vi "Queue Manager.vi"(0 "queue in":refnum<queue>, 5 "Queue States In":cluster{"Enum":T1, "Data":variant}[](array[cluster])=[{"Enum"=enum."Read GUI Pars", "Data"=variant}], 9 "Place New Element":enum16{"Back", "Front", "Replace"}(ring), 11 "Error IN":errorcluster, 12 "Ignore Errors":bool) -> (4 "queue out":refnum<queue>, 8 "Last Error":errorcluster, 15 "Error OUT":errorcluster)   [LabVIEW 2016]
uses:
  Types/State Control.ctl
  Types/Global Variables.vi
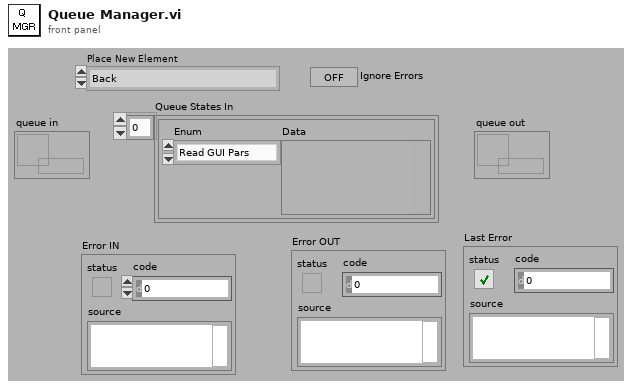
[diagram p1: front panel]
types:
  T1 = typedef "State Control.ctl" = enum16{"Startup", "Read Config File", "Initilize Optional Hardware", "Idle", "New Session", "Read GUI Pars", "Configure Hardware", "Initialize Set", "Pre-Scan", "Scan", "Post-Scan", "Exit Set", "Automated Tuning", "Manual Tuning", "Check Calibration", "Optimize RF Power", "Test Scan", "Set Oxy QA-Scan Pars", "Find Peaks", "Update from Cursors", "Flag Bad Set", "Mark transition time", "Measure Q", "Measure Noise", "Rotate Magnet", "Lock Field", "Engineering Tuning", "Zero Voltages", "Update Center Field", "Refit Data", "Open Session Data Folder", "AfterSave", "Undo Auto Update Pars", "Read from Script", "End Session", "Quit Software", "Error"}
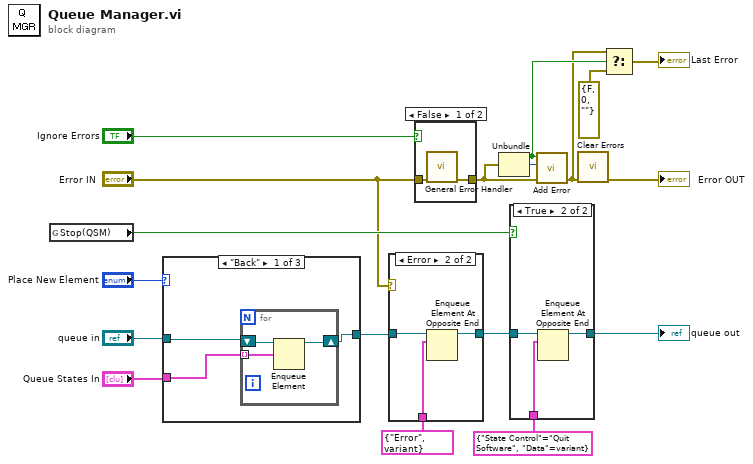
[diagram p0: block diagram]
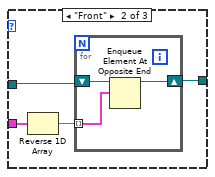
[diagram p5: hidden frame]
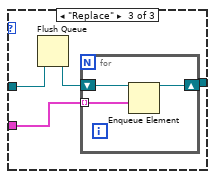
[diagram p6: hidden frame]
diagram:
  n1 = global read "Global Variables.vi" "Stop(QSM)"() -> (w10:bool)
  n2 = case shown="\"Back\"" "Place New Element" {
    tunnel: "Queue States In" -> [w19 w28 w33]
    tunnel: "queue in" -> [w21 w26 w35]
    tunnel: [w20 w25 w32] -> w17
    frame "Back" {
      n3 = for {
        shift-right: [w23] -> w20
        shift-left: w21 -> [w24]
        tunnel: w19 -> [w22] mode=indexing
        n4 = Enqueue Element(queue=w24, element=w22) -> (queue out=w23:refnum<queue>)  [unwired: 2 in, 2 out]
      }
    }
    frame "Front" {
      n5 = Reverse 1D Array(array=w28) -> (reversed array=w27:cluster{"Enum":T1, "Data":variant}[])
      n6 = for {
        tunnel: w27 -> [w30] mode=indexing
        shift-right: [w29] -> w25
        shift-left: w26 -> [w31]
        n7 = Enqueue Element At Opposite End(queue=w31, element=w30) -> (queue out=w29:refnum<queue>)  [unwired: 2 in, 2 out]
      }
    }
    frame "Replace" {
      n8 = Flush Queue(queue=w35) -> (queue out=w34:refnum<queue>)  [unwired: 1 in, 2 out]
      n9 = for {
        tunnel: w33 -> [w37] mode=indexing
        shift-right: [w36] -> w32
        shift-left: w34 -> [w38]
        n10 = Enqueue Element(queue=w38, element=w37) -> (queue out=w36:refnum<queue>)  [unwired: 2 in, 2 out]
      }
    }
  }
  n11 = case shown="Error" "Error IN" {
    tunnel: w17 -> [w39 w42]
    tunnel: [w39 w41] -> w16
    tunnel: cluster{"State Control":T1, "Data":variant} {"State Control"=enum."Error", "Data"=variant} ("element") -> [_ w40]
    frame No Error {
    }
    frame Error {
      n12 = Enqueue Element At Opposite End(queue=w42, element=w40) -> (queue out=w41:refnum<queue>)  [unwired: 2 in, 2 out]
    }
  }
  n13 = case shown="False" "Ignore Errors" {
    tunnel: [w43 w45] -> w6
    tunnel: "Error IN" -> [w44 w45]
    frame False {
      n14 = call <vilib>:"General Error Handler.vi"("error in (no error)"=w44) -> ("error out"=w43:errorcluster)  [unwired: 10 in, 4 out]
    }
    frame True {
    }
  }
  n15 = Unbundle(w6) -> ("status"=w4:bool, "code"=w8:i32)  [unwired: 1 out]
  n16 = case shown="True" w10 {
    tunnel: w16 -> [w46 w49]
    tunnel: cluster{"State Control":T1, "Data":variant} {"State Control"=enum."Quit Software", "Data"=variant} ("element") -> [_ w48]
    tunnel: [w46 w47] -> w11
    frame False {
    }
    frame True {
      n17 = Enqueue Element At Opposite End(queue=w49, element=w48) -> (queue out=w47:refnum<queue>)  [unwired: 2 in, 2 out]
    }
  }
  "queue out" <- w11
  n18 = call "Add Error.vi"("error in (no error)"=w6, "error code (0)"=w8, "error?"=w4) -> ("error out"=w3:errorcluster)  [unwired: 8 in]
  n19 = call <vilib>:"Clear Errors.vi"("error in (no error)"=w3) -> ("error out"=→"Error OUT":errorcluster)  [unwired: 5 in, 1 out]
  n20 = Select(t=w3, s=w4, f=errorcluster {"status"=FALSE, "code"=0, "source"=""}) -> (s? t:f=→"Last Error":errorcluster)
